vi "RQST Look for Response.vi"(8 "error in (no error)":errorcluster, 10 "CAN frame":T2 {"payload" format="%x"; "timestamp" format="%<%.7X\n%x>T"; "type" items=["CAN Data"=0, "CAN Remote"=1, "CAN Bus Error"=2, "J1939 Data"=192, "Delay"=224, "Log Trigger"=225, "Start Trigger"=226]; "identifier" format="%x"}, 11 "ref in":T1) -> (0 "error out":errorcluster)   [LabVIEW 2013, in "J1939.lvlib"]
uses:
  J1939.lvlib
  <vilib>/xnet/xnet.llb/XNET Frame CAN.ctl
  <vilib>/xnet/xnet.llb/XNET Frame Type CAN.ctl
  RQST Lookup Table Reference.ctl
  Frame Conversion/Convert CAN Arb ID to J1939 ID.vi
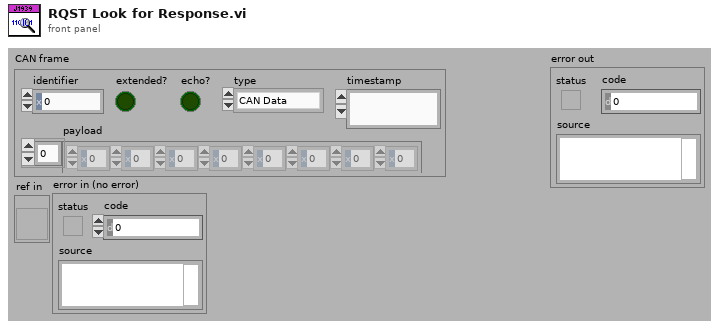
[diagram p1: front panel]
types:
  T1 = typedef "J1939.lvlib/RQST Lookup Table Reference.ctl" = refnum<vi>
  T2 = typedef "XNET Frame CAN.ctl" = cluster{"timestamp":timestamp, "payload":u8[], "identifier":u32, "type":T3, "extended?":bool, "echo?":bool}
  T3 = typedef "XNET Frame Type CAN.ctl" = u8
  T4 = typedef "J1939.lvlib/RQST Lookup Table Cluster.ctl" = cluster{"Response Q":refnum<queue>, "Request PGN":u32}
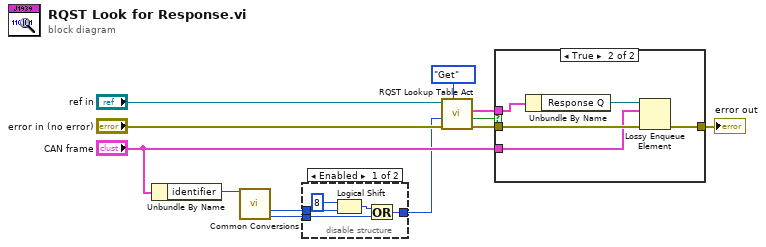
[diagram p0: block diagram]
diagram:
  n1 = Unbundle By Name("CAN frame") -> ("identifier"=w7:u32)
  n2 = call-poly "Common Conversions.vi"("Arb ID"=w7) -> ("PGN"=w8:u32, "Source Address"=w9:u8)  [unwired: 11 in, 2 out]
  n3 = disable-structure shown="Enabled" {
    disable-tunnel: w9 -> [w15 _]
    disable-tunnel: w8 -> [w14 w18]
    disable-tunnel: [w13 w18] -> w6
    frame Enabled {
      n4 = Logical Shift(y=i8 8, x=w14) -> (x << y=w17:u32)
      n5 = Or(x=w17, y=w15) -> (x .or. y?=w13:u32)
    }
    frame Disabled {
    }
  }
  n6 = call "RQST Lookup Table Act.vi"("Action"=enum16{"Initialize", "Add", "Get", "Remove"}."Get", "error in (no error)"="error in (no error)", "ID"=w6, "ref in"="ref in") -> ("error out"=w2:errorcluster, "Found?"=w4:bool, "Data"=w3:T4)  [unwired: 5 in]
  n7 = case shown="True" w4 {
    tunnel: w3 -> [_ w23]
    tunnel: w2 -> [w19 w24]
    tunnel: "CAN frame" -> [_ w21]
    tunnel: [w19 w20] -> w1
    frame False {
    }
    frame True {
      n8 = Unbundle By Name(w23) -> ("Response Q"=w22:refnum<queue>)
      n9 = Lossy Enqueue Element(queue=w22, element=w21, error in (no error)=w24) -> (error out=w20:errorcluster)  [unwired: 3 out]
    }
  }
  "error out" <- w1
